vi "Actor Core.vi"(8 "error in (no error)":errorcluster, 11 "Measurements Controller UI in":refnum<class "Measurement Controller UI.lvclass">) -> (0 "error out":errorcluster, 3 "Actor Framework.lvlib:Actor":refnum<class "Actor.lvclass">)   [LabVIEW 2015, in "Measurement Controller UI.lvclass"]
uses:
  Measurement Controller UI.lvclass
  <vilib>/ActorFramework/Actor/Actor.lvclass
  Queued Listbox/Queued Listbox.xctl
  Controls/Menu object.ctl
  Common Measurements/Common Measurements Interface/Common Measurements Interface.lvclass/Common Measurements Interface.ctl
  Mag Lab Measure Interface/Mag Lab Measure UI.lvclass/Mag Lab Measure UI.ctl
  <vilib>/ActorFramework/Actor/Actor.lvclass/Actor.ctl
  <vilib>/ActorFramework/Message Enqueuer/Message Enqueuer.lvclass/Message Enqueuer.ctl
  Mag Lab Graph/MagLabGraph.lvclass
  Mag Lab Measure Base Messages/Launch graph Msg/Launch graph Msg.lvclass/Launch graph Msg.ctl
  Mag Lab Measure Controller Messages/Start measurements Msg/Start measurements Msg.lvclass/Start measurements Msg.ctl
  Mag Lab Measure Controller Messages/Pause measurements Msg/Pause measurements Msg.lvclass/Pause measurements Msg.ctl
  Common Measurements/Common Measurements Interface/Write Time Stamp.vi
  Common Measurements/Common Measurements Interface/Write File Path 2.vi
  Common Measurements/Common Measurements Interface/Write Measurements Menu.vi
  <vilib>/ActorFramework/Message Enqueuer/Init from Existing Queue.vi
  <vilib>/ActorFramework/Message Enqueuer/Enqueue.vi
  <vilib>/ActorFramework/Message Priority Queue/Priority Enqueue.vi
  <vilib>/ActorFramework/Message Enqueuer/Message Enqueuer.lvclass
  <vilib>/ActorFramework/Stop Msg/Stop Msg.lvclass
  Mag Lab Measure Base Messages/Launch graph Msg/Launch graph Msg.lvclass
  Mag Lab Measure Controller Messages/Start measurements Msg/Start measurements Msg.lvclass
  Mag Lab Measure Controller Messages/Pause measurements Msg/Pause measurements Msg.lvclass
  Mag Lab Measure Controller Messages/Stop all measurements Msg/Stop all measurements Msg.lvclass
  Common Measurements/Common Measurements Interface/Common Measurements Interface.lvclass
  Mag Lab Measure Interface/Mag Lab Measure UI.lvclass
  Mag Lab Error Handler/Mag Lab Error Handler.lvclass
panel:
  in  "Secondary Control":T1 {"Object name" items=["Select one"]}
  in  "Primary Control":T1 {"Object name" items=["Select one"]}
  in  "Pause":bool
  in  "Repeat times":i32=-1
  in  "Time Stamp":timestamp
  in  "Stop":bool
  out "File Path":path
  in  "Graph":bool
  in  "Run":bool
  in  "Measurements":string[](xcontrol)
  out "Name":string
  in  "Parameters":cluster{"Text":string}
  out "Log":string
  in  "Exit":bool
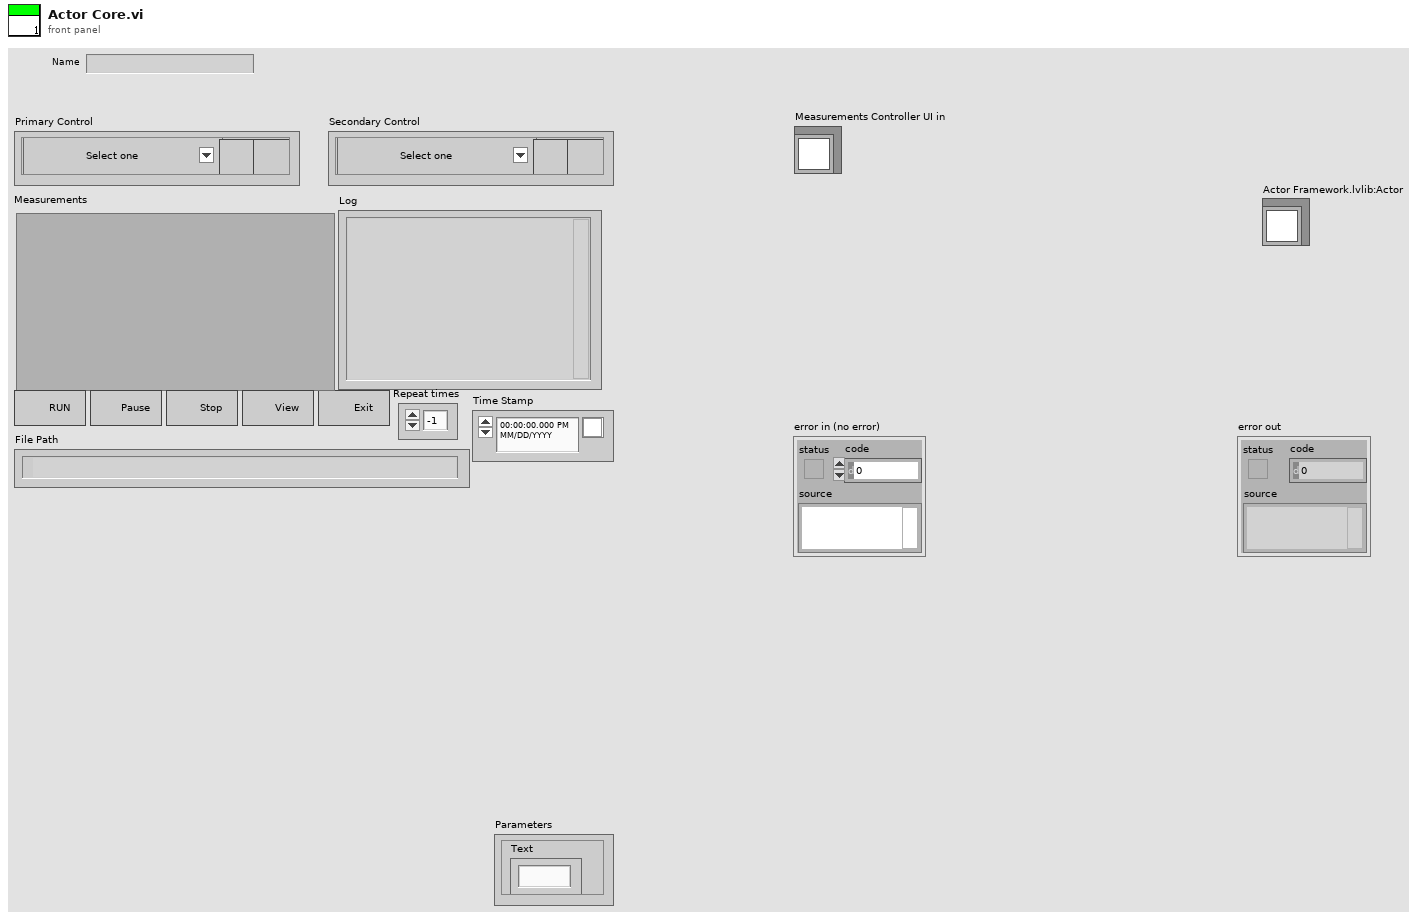
[diagram p1: front panel]
types:
  T1 = typedef "Menu object.ctl" = cluster{"Object name":u16, "Open parameters":bool, "Remove Button":bool}
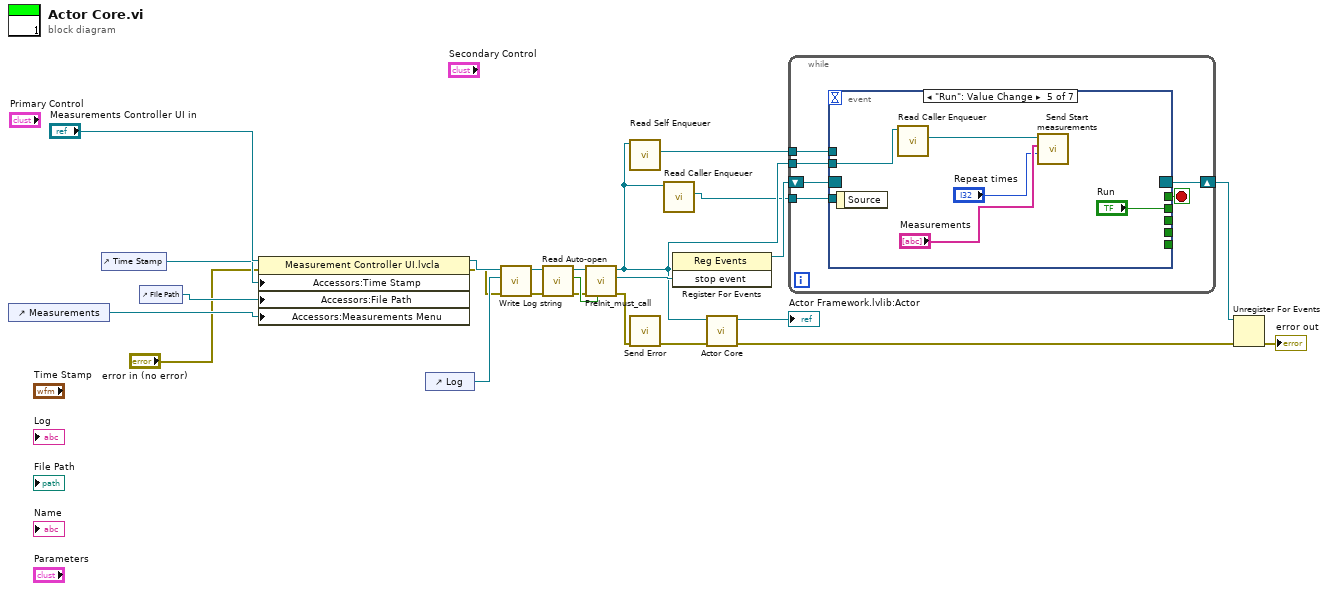
[diagram p0: block diagram]
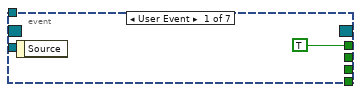
[diagram p2: hidden frame]
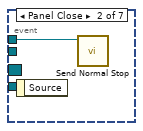
[diagram p3: hidden frame]
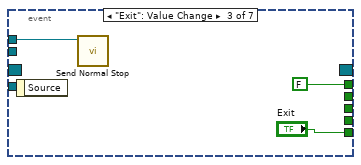
[diagram p4: hidden frame]
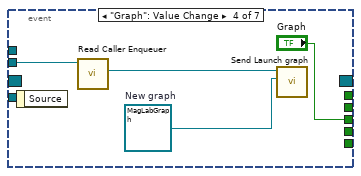
[diagram p5: hidden frame]
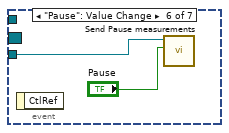
[diagram p6: hidden frame]
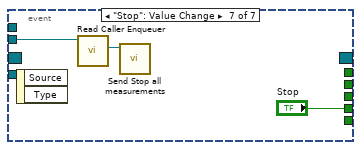
[diagram p7: hidden frame]
diagram:
  n1 = control-ref of="Measurements"() -> (w3:refnum<vi>)
  n2 = control-ref of="Time Stamp"() -> (w5:refnum<vi>)
  n3 = control-ref of="File Path"() -> (w4:refnum<vi>)
  n4 = property class="Measurement Controller UI.lvcla"(reference="Measurements Controller UI in", error in="error in (no error)", "Accessors:Time Stamp"=w5, "Accessors:File Path"=w4, "Accessors:Measurements Menu"=w3) -> (reference out=w6:refnum<class "Measurement Controller UI.lvclass">, error out=w2:errorcluster)
  n5 = control-ref of="Log"() -> (w21:refnum<vi>)
  n6 = call "Write Log string.vi"("error in (no error)"=w2, "Log string"=w21, "Mag Lab Measure Interface in"=w6) -> ("error out"=w11:errorcluster, "Mag Lab Measure Interface out"=w14:refnum<class "Measurement Controller UI.lvclass">)  [unwired: 7 in]
  n7 = call "Read Auto-open.vi"("error in (no error)"=w11, "Mag Lab Measure UI in"=w14) -> ("error out"=w10:errorcluster, "Auto-open"=w12:bool, "Mag Lab Measure UI out"=w13:refnum<class "Measurement Controller UI.lvclass">)  [unwired: 7 in]
  n8 = call-dynamic "PreInit_must_call.vi"("Open Actor Core front panel? (T)"=w12, "error in (no error)"=w10, "Mag Lab Measure Interface in"=w13) -> ("error out"=w18:errorcluster, "stop event"=w22:refnum<user-event>, "Mag Lab Measure Interface out"=w9:refnum<class "Measurement Controller UI.lvclass">)  [unwired: 6 in]
  n9 = call <vilib>:"Read Self Enqueuer.vi"("Actor"=w9) -> ("Self Enqueuer"=w20:refnum<class "Message Enqueuer.lvclass">)  [unwired: 10 in]
  n10 = call "Send Error.vi"("error in (no error)"=w18) -> ("error out"=w19:errorcluster)  [unwired: 9 in, 1 out]
  n11 = call <vilib>:"Read Caller Enqueuer.vi"("Actor"=w9) -> ("Caller Enqueuer"=w8:refnum<class "Message Enqueuer.lvclass">)  [unwired: 10 in]
  n12 = register-events(w22) -> (reference out=w23:refnum<event-registration>)  [unwired: 2 in, 1 out]
  n13 = call-parent "Actor Core.vi"("error in (no error)"=w19, "Common Measurements Interface in"=w9) -> ("error out"=w15:errorcluster, "Actor Framework.lvlib:Actor"=→"Actor Framework.lvlib:Actor":refnum<class "Actor.lvclass">)  [unwired: 8 in]
  n14 = while {
    tunnel: w20 -> [w28]
    shift-right: [w27] -> w16
    shift-left: w23 -> [w29]
    tunnel: w9 -> [w26]
    tunnel: w8 -> [w25]
    stop <- w30 stop-if-true
    n15 = event shown="[4] \"Run\": Value Change" {
      selector: w29 -> [_ _ _ _ _ _ _]
      dyn-events: [_ _ _ _ _ _ _] -> w27
      timeout: _ -> [_ _ _ _ _ _ _]
      tunnel: [TRUE _ FALSE _ _ _ _] -> w30
      tunnel: w28 -> [_ w32 w33 _ _ _ _]
      tunnel: [_ _ "Exit" _ _ _ _] -> _
      tunnel: [_ _ _ _ "Run" _ _] -> _
      tunnel: w26 -> [_ _ _ w39 w43 _ w48]
      tunnel: [_ _ _ "Graph" _ _ _] -> _
      tunnel: [_ _ _ _ _ _ "Stop"] -> _
      tunnel: w25 -> [_ _ _ _ _ w45 _]
      event User Event {
        n16 = event-data() -> ()  [unwired: 1 in, 1 out]
      }
      event Panel Close {
        n17 = event-data() -> ()  [unwired: 1 in, 1 out]
        n18 = call <vilib>:"Send Normal Stop.vi"("Message Enqueuer"=w32) -> ()  [unwired: 10 in, 1 out]
      }
      event "Exit": Value Change {
        n19 = event-data() -> ()  [unwired: 1 in, 1 out]
        n20 = call <vilib>:"Send Normal Stop.vi"("Message Enqueuer"=w33) -> ()  [unwired: 10 in, 1 out]
      }
      event "Graph": Value Change {
        w37 = refnum<class "MagLabGraph.lvclass"> refnum  # New graph
        n21 = event-data() -> ()  [unwired: 1 in, 1 out]
        n22 = call <vilib>:"Read Caller Enqueuer.vi"("Actor"=w39) -> ("Caller Enqueuer"=w38:refnum<class "Message Enqueuer.lvclass">)  [unwired: 10 in]
        n23 = call "Send Launch graph.vi"("MagLabGraph.lvclass"=w37, "Message Enqueuer"=w38) -> ()  [unwired: 8 in, 2 out]
      }
      event "Run": Value Change {
        n24 = event-data() -> ()  [unwired: 1 in, 1 out]
        n25 = call <vilib>:"Read Caller Enqueuer.vi"("Actor"=w43) -> ("Caller Enqueuer"=w42:refnum<class "Message Enqueuer.lvclass">)  [unwired: 10 in]
        n26 = call "Send Start measurements.vi"("Repeat times"="Repeat times", "Measurements"="Measurements", "Message Enqueuer"=w42) -> ()  [unwired: 7 in, 2 out]
      }
      event "Pause": Value Change {
        n27 = event-data() -> ()  [unwired: 1 in, 1 out]
        n28 = call "Send Pause measurements.vi"("Pause"="Pause", "Message Enqueuer"=w45) -> ()  [unwired: 8 in, 2 out]
      }
      event "Stop": Value Change {
        n29 = event-data() -> ()  [unwired: 1 in, 2 out]
        n30 = call <vilib>:"Read Caller Enqueuer.vi"("Actor"=w48) -> ("Caller Enqueuer"=w47:refnum<class "Message Enqueuer.lvclass">)  [unwired: 10 in]
        n31 = call "Send Stop all measurements.vi"("Message Enqueuer"=w47) -> ()  [unwired: 9 in, 2 out]
      }
    }
  }
  n32 = Unregister For Events(event registration refnum=w16, error in=w15) -> (error out=→"error out":errorcluster)
